vi "TAT_Com_PLC.vi"() -> ()   [LabVIEW 2017]
uses:
  <vilib>/NI/Modbus Library/API/Wrapper/Create TCP Master.vi
  Global/Global 1.vi
  <vilib>/NI/Modbus Library/API/Master/Modbus Master.lvclass
  <vilib>/NI/Modbus Library/API/Wrapper/API Main.lvlib
panel:
  out "register values":u16[](array[numeric])
  out "error out 3":errorcluster
  out "Read set 2":u16[](array[numeric])
  out "boolean out 2":bool[](array[boolean])
  out "Write to PLC 2":bool[](array[boolean])
  out "Scanned Value D6000":string
  out "boolean out":bool[](array[boolean])
  out "Scanned Value D6000":string
  in  "stop 2":bool
  out "PLC STATUS 2":bool
  in  "error in 2":errorcluster
  out "error out 2":errorcluster
  out "Write to PLC":bool[](array[boolean])
  out "error out":errorcluster
  out "Read set 1":u16[](array[numeric])
  out "PLC STATUS station 1":bool
  in  "error in":errorcluster
  in  "stop":bool
  # "Station 1"
  # "CYCLE TIME\nAMBIENT TEMP\nBLINKER CURRENT OK\nTEMP SENSOR OK\nPART OK COUNT\nPART NOK COUNT\nFAULT BIT\nVARIENT\nHOUR\nMINUTE\nSECOND\nDAY\nMONTH\nYEAR\nSERIAL NUMBER\nShift\nAVM\nTS\nIV3"
  # "2590"
  # "2338"
  # "4350"
  # "BLINKER CURRENT OK\nTEMP SENSOR OK\nAVM OK\nIV3 CAMERA OK SIGNAL\nCYCLE COMPLETE\nCYCLE START (RUN CY)\nCYCLE STOP\nSCAN BYPASS\nRQS TO TCO READ SCN DTA"
  # "7"
  # "15"
  # "SCAN OK\nSCAN NG \nSoftware on Bit\nRQST FRM TCO REST SCN DT"
  # "2588"
  # "2"
  # "Station 2"
  # "1 CYCLE TIME--7196\n\n\n\n\n\n7 FAULT BIT ----4356\nVARIENT\nHOUR\nMINUTE\nSECOND\nDAY\nMONTH\nYEAR\nSERIAL NUMBER\nShift\n17 POWER FOLD ACTUATO--D6061\nGLASS ACTUATOR 1 &2"
  # "SCAN BYPASS---2598---M550\nRQS TO TCO READ SCAN DATA \nsql bypass\nCYCLE START (RUNNING CYCLE)\nCYCLE  STOP\nCYCLE COMPLETE\n--45325\nby pass station 1 Bit\nStation 1 valid BIT"
  # "SCAN OK\nSCAN NG \nSoftware on Bit\nRQST FRM TCO REST SCN"
  # "POWER FOLD CURENT 6296\nGLASS ACTUATOR CURANT 1 MA 6297\nGLASS ACTUATOR CURANT 2 MA 6298\nGLASS PUL TEST  D2206 6302\n\nSKY  D2208 6304\n\nGROUND  6306\n\nINTERNAL(DEG)  6308\n\nEXTERNAL(DEG)  6310"
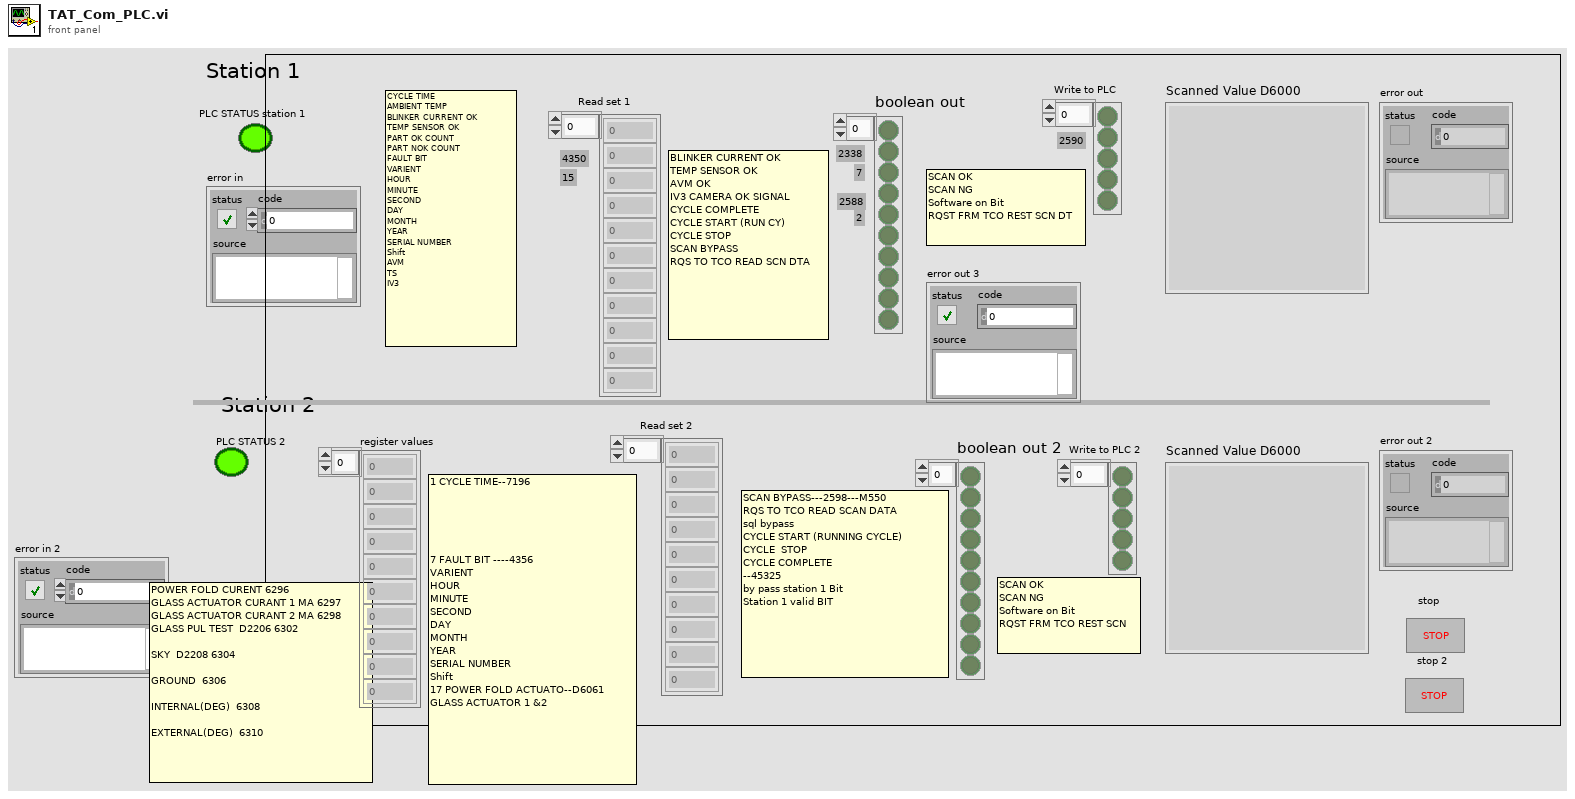
[diagram p1: front panel]
types:
  T1 = enum32{"invalid app kind", "Development System", "Run Time System", "Student Edition", "Embedded LabVIEW", "Evaluation", "Custom"}
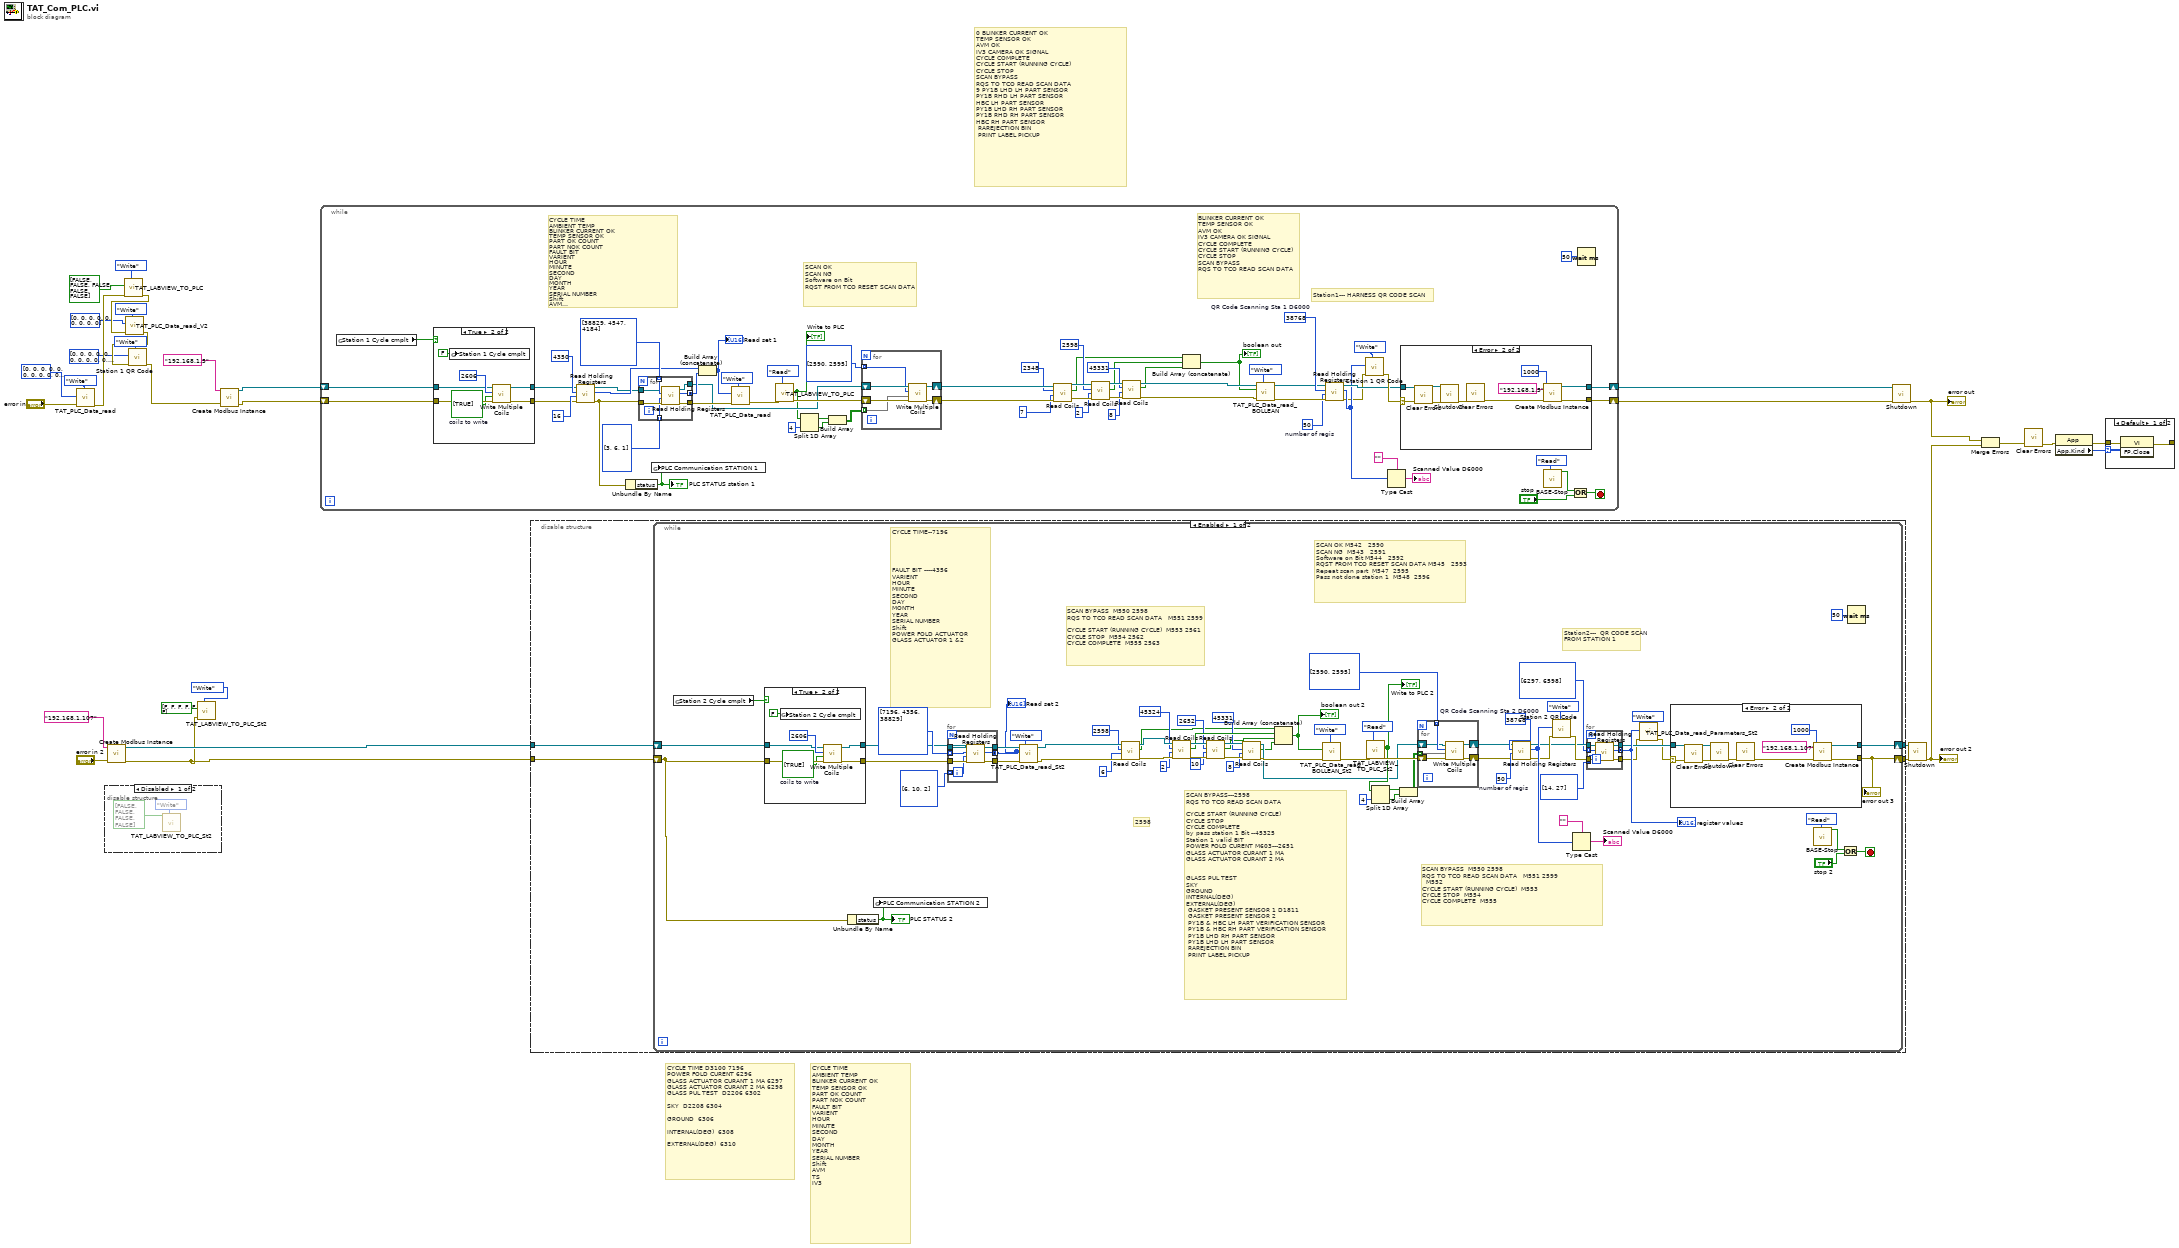
[diagram p0: block diagram]
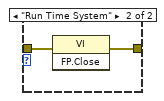
[diagram p8: hidden frame]
diagram:
  # "0 BLINKER CURRENT OK\nTEMP SENSOR OK\nAVM OK\nIV3 CAMERA OK SIGNAL\nCYCLE COMPLETE\nCYCLE START (RUNNING CYCLE)\nCYCLE STOP\nSCAN BYPASS\nRQS TO TCO READ SCAN DATA \n9 PY1B LHD LH PART SENSOR\nPY1B RHD LH PART SENSOR  \nHBC LH PART SENSOR  \nPY1B LHD RH PART SENSOR  \nPY1B RHD RH PART SENSOR  \nHBC RH PART SENSOR  \n RAREJECTION BIN\n PRINT LABEL PICKUP"
  # "CYCLE TIME\nAMBIENT TEMP\nBLINKER CURRENT OK\nTEMP SENSOR OK\nPART OK COUNT\nPART NOK COUNT\nFAULT BIT\nVARIENT\nHOUR\nMINUTE\nSECOND\nDAY\nMONTH\nYEAR\nSERIAL NUMBER\nShift\nAVM\nTS\nIV3"
  # "CYCLE TIME D3100 7196\nPOWER FOLD CURENT 6296\nGLASS ACTUATOR CURANT 1 MA 6297\nGLASS ACTUATOR CURANT 2 MA 6298\nGLASS PUL TEST  D2206 6302\n\nSKY  D2208 6304\n\nGROUND  6306\n\nINTERNAL(DEG)  6308\n\nEXTERNAL(DEG)  6310"
  n1 = call "TAT_PLC_Data_read.vi"("Enum"=enum16{"Read", "Write"}."Write", "error in (no error)"="error in", "Array"=u16[] [0, 0, 0, 0, 0, 0, 0, 0, 0, 0, 0, 0, 0, 0, 0, 0, 0, 0, 0, 0, 0] ("Array 3")) -> ("error out"=w22:errorcluster)  [unwired: 7 in, 1 out]
  n2 = disable-structure shown="Disabled" {
    frame Disabled {
      n3 = call "TAT_LABVIEW_TO_PLC_St2.vi"("Enum"=enum16{"Read", "Write"}."Write", "Array"=bool[] [FALSE, FALSE, FALSE, FALSE]) -> ()  [unwired: 8 in, 2 out]
    }
    frame Enabled {
    }
  }
  n4 = call-poly <vilib>:"Create Modbus Instance.vi"("error in"="error in 2", "address"="192.168.1.107") -> ("error out"=w1:errorcluster, "TCP master instance"=w14:refnum<class "Modbus Master.lvclass">)  [unwired: 8 in]
  n5 = call "TAT_LABVIEW_TO_PLC.vi"("Enum"=enum16{"Read", "Write"}."Write", "error in (no error)"=w22, "Array"=bool[] [FALSE, FALSE, FALSE, FALSE, FALSE]) -> ("error out"=w17:errorcluster)  [unwired: 7 in, 1 out]
  n6 = call "TAT_PLC_Data_read_V2.vi"("Enum"=enum16{"Read", "Write"}."Write", "error in (no error)"=w17, "Array"=u16[] [0, 0, 0, 0, 0, 0, 0, 0, 0] ("Array 3")) -> ("error out"=w10:errorcluster)  [unwired: 7 in, 1 out]
  n7 = call "Station 1 QR Code.vi"("Enum"=enum16{"Read", "Write"}."Write", "error in (no error)"=w10, "Array"=u16[] [0, 0, 0, 0, 0, 0, 0, 0, 0, 0, 0, 0, 0, 0, 0, 0, 0, 0, 0, 0, 0, 0, 0, 0, 0, 0, 0, 0, 0, 0, 0, 0, 0, 0, 0, 0, 0, 0, 0, 0, 0, 0, 0, 0, 0, 0, 0, 0, 0, 0, 0, 0, 0, 0, 0, 0, 0, 0, 0, 0, 0] ("Array 3")) -> ("error out"=w11:errorcluster)  [unwired: 7 in, 1 out]
  n8 = call "TAT_LABVIEW_TO_PLC_St2.vi"("Enum"=enum16{"Read", "Write"}."Write", "error in (no error)"=w1, "Array"=bool[] [FALSE, FALSE, FALSE, FALSE, FALSE, FALSE]) -> ()  [unwired: 7 in, 2 out]
  n9 = call-poly <vilib>:"Create Modbus Instance.vi"("error in"=w11, "address"="192.168.1.5") -> ("error out"=w27:errorcluster, "TCP master instance"=w26:refnum<class "Modbus Master.lvclass">)  [unwired: 8 in]
  n10 = while {
    shift-right: [w95] -> w31
    shift-left: w26 -> [w52]
    shift-right: [w94] -> w30
    shift-left: w27 -> [w54]
    stop <- w96 stop-if-true
    w76 = u16 50  # number of regis
    w77 = u16 38768  # QR Code Scanning Sta 1 D6000
    # "SCAN OK\nSCAN NG \nSoftware on Bit\nRQST FROM TCO RESET SCAN DATA"
    # "BLINKER CURRENT OK\nTEMP SENSOR OK\nAVM OK\nIV3 CAMERA OK SIGNAL\nCYCLE COMPLETE\nCYCLE START (RUNNING CYCLE)\nCYCLE STOP\nSCAN BYPASS\nRQS TO TCO READ SCAN DATA"
    # "Station1--- HARNESS QR CODE SCAN"
    # "CYCLE TIME\nAMBIENT TEMP\nBLINKER CURRENT OK\nTEMP SENSOR OK\nPART OK COUNT\nPART NOK COUNT\nFAULT BIT\nVARIENT\nHOUR\nMINUTE\nSECOND\nDAY\nMONTH\nYEAR\nSERIAL NUMBER\nShift\nAVM\nTS\nIV3 CAMERA"
    n11 = global read "Global 1.vi" "Station 1 Cycle cmplt"() -> (w55:bool)
    n12 = case shown="True" w55 {
      tunnel: w52 -> [w98 w105]
      tunnel: [w98 w104] -> w51
      tunnel: w54 -> [w99 w103]
      tunnel: [w99 w102] -> w53
      frame False {
      }
      frame True {
        w100 = bool[] [TRUE]  # coils to write
        n13 = global write "Global 1.vi" "Station 1 Cycle cmplt"(FALSE) -> ()
        n14 = call-dynamic "Write Multiple Coils.vi"("error in"=w103, "coils to write"=w100, "starting address"=2606 ("CYCLE TIME"), "Modbus master in"=w105) -> ("error out"=w102:errorcluster, "Modbus master out"=w104:refnum<class "Modbus Master.lvclass">)  [unwired: 6 in]
      }
    }
    n15 = call-dynamic "Read Holding Registers.vi"("error in"=w53, "number of inputs"=u16 16, "starting address"=u16 4350 ("starting address 2"), "Modbus master in"=w51) -> ("error out"=w72:errorcluster, "register values"=w66:u16[], "Modbus master out"=w64:refnum<class "Modbus Master.lvclass">)  [unwired: 5 in]
    n16 = Unbundle By Name(w72) -> ("status"=w84:bool)
    "PLC STATUS station 1" <- w84
    n17 = for {
      tunnel: u16[] [38829, 4547, 4184] ("starting address 2") -> [w118] mode=indexing
      tunnel: u16[] [3, 6, 1] ("number of inputs") -> [w117] mode=indexing
      tunnel: [w115] -> w65 mode=concatenating
      tunnel: w64 -> [w114]
      tunnel: [w113] -> w63
      tunnel: w72 -> [w119]
      tunnel: [w116] -> w68
      n18 = call-dynamic "Read Holding Registers.vi"("error in"=w119, "number of inputs"=w117, "starting address"=w118, "Modbus master in"=w114) -> ("error out"=w116:errorcluster, "register values"=w115:u16[], "Modbus master out"=w113:refnum<class "Modbus Master.lvclass">)  [unwired: 5 in]
    }
    n19 = global write "Global 1.vi" "PLC Communication STATION 1"(w84) -> ()
    n20 = Build Array (concatenate)(w66, w65) -> (w62:u16[])
    "Read set 1" <- w62
    n21 = call "TAT_PLC_Data_read.vi"("Enum"=enum16{"Read", "Write"}."Write", "error in (no error)"=w68, "Array"=w62) -> ("error out"=w67:errorcluster)  [unwired: 7 in, 1 out]
    n22 = call "TAT_LABVIEW_TO_PLC.vi"("Enum"=enum16{"Read", "Write"}."Read", "error in (no error)"=w67) -> ("error out"=w89:errorcluster, "Array 2"=w60:bool[])  [unwired: 8 in]
    "Write to PLC" <- w60
    n23 = Split 1D Array(array=w60, index=4) -> (first subarray=w59:bool[], second subarray=w58:bool[])
    n24 = Build Array(w59, w58) -> (w57:bool[][])
    n25 = for {
      tunnel: w57 -> [w111] mode=indexing
      shift-right: [w110] -> w86
      shift-left: w89 -> [w112]
      shift-right: [w109] -> w85
      shift-left: w63 -> [w108]
      tunnel: u16[] [2590, 2595] ("starting address") -> [w107] mode=indexing
      n26 = call-dynamic "Write Multiple Coils.vi"("error in"=w112, "coils to write"=w111, "starting address"=w107, "Modbus master in"=w108) -> ("error out"=w110:errorcluster, "Modbus master out"=w109:refnum<class "Modbus Master.lvclass">)  [unwired: 6 in]
    }
    n27 = call-dynamic "Read Coils.vi"("error in"=w86, "number of inputs"=7, "starting address"=2348, "Modbus master in"=w85) -> ("error out"=w49:errorcluster, "coils"=w38:bool[], "Modbus master out"=w50:refnum<class "Modbus Master.lvclass">)  [unwired: 5 in]
    n28 = call-dynamic "Read Coils.vi"("error in"=w49, "number of inputs"=2, "starting address"=2598, "Modbus master in"=w50) -> ("error out"=w47:errorcluster, "coils"=w37:bool[], "Modbus master out"=w48:refnum<class "Modbus Master.lvclass">)  [unwired: 5 in]
    n29 = call-dynamic "Read Coils.vi"("error in"=w47, "number of inputs"=8, "starting address"=45331, "Modbus master in"=w48) -> ("error out"=w45:errorcluster, "coils"=w36:bool[], "Modbus master out"=w46:refnum<class "Modbus Master.lvclass">)  [unwired: 5 in]
    n30 = Build Array (concatenate)(w38, w37, w36) -> (w35:bool[])
    "boolean out" <- w35
    n31 = call "TAT_PLC_Data_read_BOLLEAN.vi"("Enum"=enum16{"Read", "Write"}."Write", "error in (no error)"=w45, "Array"=w35) -> ("error out"=w79:errorcluster)  [unwired: 7 in, 1 out]
    n32 = call-dynamic "Read Holding Registers.vi"("error in"=w79, "number of inputs"=w76, "starting address"=w77, "Modbus master in"=w46) -> ("error out"=w73:errorcluster, "register values"=w74:u16[], "Modbus master out"=w78:refnum<class "Modbus Master.lvclass">)  [unwired: 5 in]
    n33 = call "Station 1 QR Code.vi"("Enum"=enum16{"Read", "Write"}."Write", "error in (no error)"=w73, "Array"=w74) -> ("error out"=w80:errorcluster)  [unwired: 7 in, 1 out]
    n34 = Type Cast(type="", x=w74) -> (*(type *) &x=→"Scanned Value D6000":string)
    n35 = case shown="Error" w80 {
      selector: w80 -> [w120 w130]
      tunnel: w78 -> [w121 w128]
      tunnel: [w121 w124] -> w95
      tunnel: [w120 w123] -> w94
      frame No Error {
      }
      frame Error {
        n36 = call <vilib>:"Clear Errors.vi"("error in (no error)"=w130) -> ("error out"=w129:errorcluster)  [unwired: 5 in, 1 out]
        n37 = call-dynamic "Shutdown.vi"("error in"=w129, "Modbus master in"=w128) -> ("error out"=w127:errorcluster)  [unwired: 9 in]
        n38 = call <vilib>:"Clear Errors.vi"("error in (no error)"=w127) -> ("error out"=w125:errorcluster)  [unwired: 5 in, 1 out]
        n39 = call-poly <vilib>:"Create Modbus Instance.vi"("error in"=w125, "connect timeout ms"=1000, "address"="192.168.1.5") -> ("error out"=w123:errorcluster, "TCP master instance"=w124:refnum<class "Modbus Master.lvclass">)  [unwired: 7 in]
      }
    }
    n40 = call "BASE-Stop.vi"("Enum"=enum16{"Read", "Write"}."Read") -> ("Stop"=w87:bool)  [unwired: 10 in]
    n41 = Or(x=w87, y="stop") -> (x .or. y?=w96:bool)
    n42 = Wait (ms)(milliseconds to wait=u32 50) -> ()  [unwired: 1 out]
  }
  n43 = disable-structure shown="Enabled" {
    disable-tunnel: w14 -> [w134 w244]
    disable-tunnel: w1 -> [w133 w245]
    disable-tunnel: [w132 w245] -> w4
    disable-tunnel: [w131 w244] -> w13
    frame Enabled {
      n44 = while {
        shift-right: [w201] -> w131
        shift-left: w134 -> [w160]
        shift-right: [w200] -> w132
        shift-left: w133 -> [w158]
        stop <- w202 stop-if-true
        w189 = u16 50  # number of regis
        w188 = u16 38768  # QR Code Scanning Sta 2 D6000
        # "SCAN BYPASS\t\tM550\t2598\nRQS TO TCO READ SCAN DATA \t\tM551\t2599\n\t\tM552\t\nCYCLE START (RUNNING CYCLE)\t\tM553\t\nCYCLE STOP\t\tM554\t\nCYCLE COMPLETE\t\tM555"
        # "SCAN OK\tM542\t\t\t2590\nSCAN NG \tM543\t\t\t2591\nSoftware on Bit\tM544\t\t\t2592\nRQST FROM TCO RESET SCAN DATA\tM545\t\t\t2593\nRepeat scan part\t\tM547\t\t2595\nPass not done station 1\t\tM548\t\t2596"
        # "SCAN BYPASS\t\tM550\t2598\nRQS TO TCO READ SCAN DATA \t\tM551\t2599\n\nCYCLE START (RUNNING CYCLE)\t\tM553\t2561\nCYCLE STOP\t\tM554\t2562\nCYCLE COMPLETE\t\tM555\t2563"
        # "CYCLE TIME--7196\n\n\n\n\n\nFAULT BIT ----4356\nVARIENT\nHOUR\nMINUTE\nSECOND\nDAY\nMONTH\nYEAR\nSERIAL NUMBER\nShift\nPOWER FOLD ACTUATOR\nGLASS ACTUATOR 1 &2"
        # "SCAN BYPASS---2598\nRQS TO TCO READ SCAN DATA \n\nCYCLE START (RUNNING CYCLE)\nCYCLE STOP\nCYCLE COMPLETE\nby pass station 1 Bit --45325\nStation 1 valid BIT\nPOWER FOLD CURENT M603---2651\nGLASS ACTUATOR CURANT 1 MA\nGLASS ACTUATOR CURANT 2 MA\n\n\nGLASS PUL TEST\nSKY \nGROUND\nINTERNAL(DEG)\nEXTERNAL(DEG)\n GASKET PRESENT SENSOR 1 D1811\n GASKET PRESENT SENSOR 2\n PY1B & HBC LH PART VERIFICATION SENSOR\n PY1B & HBC RH PART VERIFICATION SENSOR\n PY1B LHD RH PART SENSOR\n PY1B LHD LH PART SENSOR\n RAREJECTION BIN\n PRINT LABEL PICKUP"
        # "2598"
        # "Station2---  QR CODE SCAN FROM STATION 1"
        n45 = global read "Global 1.vi" "Station 2 Cycle cmplt"() -> (w156:bool)
        n46 = case shown="True" w156 {
          tunnel: w160 -> [w204 w211]
          tunnel: [w204 w210] -> w159
          tunnel: w158 -> [w205 w209]
          tunnel: [w205 w208] -> w157
          frame False {
          }
          frame True {
            w206 = bool[] [TRUE]  # coils to write
            n47 = global write "Global 1.vi" "Station 2 Cycle cmplt"(FALSE) -> ()
            n48 = call-dynamic "Write Multiple Coils.vi"("error in"=w209, "coils to write"=w206, "starting address"=2606 ("CYCLE TIME"), "Modbus master in"=w211) -> ("error out"=w208:errorcluster, "Modbus master out"=w210:refnum<class "Modbus Master.lvclass">)  [unwired: 6 in]
          }
        }
        n49 = Unbundle By Name(w158) -> ("status"=w196:bool)
        "PLC STATUS 2" <- w196
        n50 = global write "Global 1.vi" "PLC Communication STATION 2"(w196) -> ()
        n51 = for {
          tunnel: w159 -> [w232]
          tunnel: [w231] -> w177
          tunnel: [w230] -> w175
          tunnel: w157 -> [w229]
          tunnel: u16[] [6, 10, 2] ("number of inputs") -> [w228] mode=indexing
          tunnel: u16[] [7196, 4356, 38829] ("CYCLE TIME") -> [w227] mode=indexing
          tunnel: [w226] -> w176 mode=concatenating
          n52 = call-dynamic "Read Holding Registers.vi"("error in"=w229, "number of inputs"=w228, "starting address"=w227, "Modbus master in"=w232) -> ("error out"=w230:errorcluster, "register values"=w226:u16[], "Modbus master out"=w231:refnum<class "Modbus Master.lvclass">)  [unwired: 5 in]
        }
        "Read set 2" <- w176
        n53 = call "TAT_PLC_Data_read_St2.vi"("Enum"=enum16{"Read", "Write"}."Write", "error in (no error)"=w175, "Array"=w176) -> ("error out"=w195:errorcluster)  [unwired: 7 in, 1 out]
        n54 = call-dynamic "Read Coils.vi"("error in"=w195, "number of inputs"=u16 6, "starting address"=u16 2598, "Modbus master in"=w177) -> ("error out"=w154:errorcluster, "coils"=w138:bool[], "Modbus master out"=w155:refnum<class "Modbus Master.lvclass">)  [unwired: 5 in]
        n55 = call-dynamic "Read Coils.vi"("error in"=w154, "number of inputs"=u16 2, "starting address"=45324, "Modbus master in"=w155) -> ("error out"=w152:errorcluster, "coils"=w145:bool[], "Modbus master out"=w153:refnum<class "Modbus Master.lvclass">)  [unwired: 5 in]
        n56 = call-dynamic "Read Coils.vi"("error in"=w152, "number of inputs"=10, "starting address"=2652, "Modbus master in"=w153) -> ("error out"=w150:errorcluster, "coils"=w137:bool[], "Modbus master out"=w151:refnum<class "Modbus Master.lvclass">)  [unwired: 5 in]
        n57 = call-dynamic "Read Coils.vi"("error in"=w150, "number of inputs"=8, "starting address"=45331, "Modbus master in"=w151) -> ("error out"=w149:errorcluster, "coils"=w136:bool[], "Modbus master out"=w148:refnum<class "Modbus Master.lvclass">)  [unwired: 5 in]
        n58 = Build Array (concatenate)(w138, w145, w137, w136) -> (w135:bool[])
        "boolean out 2" <- w135
        n59 = call "TAT_PLC_Data_read_BOLLEAN_St2.vi"("Enum"=enum16{"Read", "Write"}."Write", "error in (no error)"=w149, "Array"=w135) -> ("error out"=w181:errorcluster)  [unwired: 7 in, 1 out]
        n60 = call "TAT_LABVIEW_TO_PLC_St2.vi"("Enum"=enum16{"Read", "Write"}."Read", "error in (no error)"=w181) -> ("error out"=w185:errorcluster, "Array 2"=w162:bool[])  [unwired: 8 in]
        "Write to PLC 2" <- w162
        n61 = Split 1D Array(array=w162, index=4) -> (first subarray=w163:bool[], second subarray=w165:bool[])
        n62 = Build Array(w163, w165) -> (w161:bool[][])
        n63 = for {
          tunnel: w161 -> [w218] mode=indexing
          tunnel: u16[] [2590, 2595] ("starting address") -> [w217] mode=indexing
          shift-right: [w215] -> w183
          shift-left: w185 -> [w216]
          shift-right: [w214] -> w182
          shift-left: w148 -> [w213]
          n64 = call-dynamic "Write Multiple Coils.vi"("error in"=w216, "coils to write"=w218, "starting address"=w217, "Modbus master in"=w213) -> ("error out"=w215:errorcluster, "Modbus master out"=w214:refnum<class "Modbus Master.lvclass">)  [unwired: 6 in]
        }
        n65 = call-dynamic "Read Holding Registers.vi"("error in"=w183, "number of inputs"=w189, "starting address"=w188, "Modbus master in"=w182) -> ("error out"=w190:errorcluster, "register values"=w191:u16[], "Modbus master out"=w172:refnum<class "Modbus Master.lvclass">)  [unwired: 5 in]
        n66 = call "Station 2 QR Code.vi"("Enum"=enum16{"Read", "Write"}."Write", "error in (no error)"=w190, "Array"=w191) -> ("error out"=w174:errorcluster)  [unwired: 7 in, 1 out]
        n67 = Type Cast(type="", x=w191) -> (*(type *) &x=→"Scanned Value D6000":string)
        n68 = for {
          tunnel: [w224] -> w173 mode=concatenating
          tunnel: u16[] [6297, 6598] ("starting address") -> [w220] mode=indexing
          tunnel: u16[] [14, 27] ("number of inputs") -> [w219] mode=indexing
          tunnel: w172 -> [w223]
          tunnel: [w222] -> w171
          tunnel: w174 -> [w225]
          tunnel: [w221] -> w170
          n69 = call-dynamic "Read Holding Registers.vi"("error in"=w225, "number of inputs"=w219, "starting address"=w220, "Modbus master in"=w223) -> ("error out"=w221:errorcluster, "register values"=w224:u16[], "Modbus master out"=w222:refnum<class "Modbus Master.lvclass">)  [unwired: 5 in]
        }
        "register values" <- w173
        n70 = call "TAT_PLC_Data_read_Parameters_St2.vi"("Enum"=enum16{"Read", "Write"}."Write", "error in (no error)"=w170, "Array"=w173) -> ("error out"=w169:errorcluster)  [unwired: 7 in, 1 out]
        n71 = case shown="Error" w169 {
          selector: w169 -> [w233 w243]
          tunnel: w171 -> [w234 w241]
          tunnel: [w234 w237] -> w201
          tunnel: [w233 w236] -> w200
          frame No Error {
          }
          frame Error {
            n72 = call <vilib>:"Clear Errors.vi"("error in (no error)"=w243) -> ("error out"=w242:errorcluster)  [unwired: 5 in, 1 out]
            n73 = call-dynamic "Shutdown.vi"("error in"=w242, "Modbus master in"=w241) -> ("error out"=w240:errorcluster)  [unwired: 9 in]
            n74 = call <vilib>:"Clear Errors.vi"("error in (no error)"=w240) -> ("error out"=w238:errorcluster)  [unwired: 5 in, 1 out]
            n75 = call-poly <vilib>:"Create Modbus Instance.vi"("error in"=w238, "connect timeout ms"=1000, "address"="192.168.1.107") -> ("error out"=w236:errorcluster, "TCP master instance"=w237:refnum<class "Modbus Master.lvclass">)  [unwired: 7 in]
          }
        }
        "error out 3" <- w200
        n76 = call "BASE-Stop.vi"("Enum"=enum16{"Read", "Write"}."Read") -> ("Stop"=w197:bool)  [unwired: 10 in]
        n77 = Or(x=w197, y="stop 2") -> (x .or. y?=w202:bool)
        n78 = Wait (ms)(milliseconds to wait=u32 50) -> ()  [unwired: 1 out]
      }
    }
    frame Disabled {
    }
  }
  n79 = call-dynamic "Shutdown.vi"("error in"=w30, "Modbus master in"=w31) -> ("error out"=w7:errorcluster)  [unwired: 9 in]
  "error out" <- w7
  n80 = call-dynamic "Shutdown.vi"("error in"=w4, "Modbus master in"=w13) -> ("error out"=w6:errorcluster)  [unwired: 9 in]
  "error out 2" <- w6
  n81 = Merge Errors(w7, w6) -> (w5:errorcluster)
  n82 = call <vilib>:"Clear Errors.vi"("error in (no error)"=w5) -> ("error out"=w19:errorcluster)  [unwired: 5 in, 1 out]
  n83 = property class="App"(error in=w19) -> (error out=w28:errorcluster, "App.Kind"=w29:T1)  [unwired: 1 in, 1 out]
  n84 = case shown="Default" w29 {
    tunnel: w28 -> [w247 w249]
    tunnel: [w246 w248] -> _
    frame Default {
      n85 = invoke class="VI" method="FP.Close"(error in=w247) -> (error out=w246:errorcluster)  [unwired: 2 in, 2 out]
    }
    frame "Run Time System" {
      n86 = invoke class="VI" method="FP.Close"(error in=w249) -> (error out=w248:errorcluster)  [unwired: 2 in, 2 out]
    }
  }
